vi "filter-scan-data-by-idx.vi"(9 "scan-idx-as-double":dbl=-1.0 format="%#_13g", 10 "meta-column-idx":i32=4, 11 "data-in":dbl[][](array[numeric])=[[1.0, 0.0, 0.0, 0.0, 1.0], [2.0, 0.0, 0.0, 0.0, 1.0], [3.0, 0.0, 0.0, 0.0, -1.0], [4.0, 0.0, 0.0, 0.0, -1.0], [5.0, 0.0, 0.0, 0.0, -1.0], [6.0, 0.0, 0.0, 0.0, -1.0], [7.0, 0.0, 0.0, 0.0, -1.0], [8.0, 0.0, 0.0, 0.0, -1.0], [9.0, 0.0, 0.0, 0.0, -1.0], [10.0, 0.0, 0.0, 0.0, 1.0], [11.0, 0.0, 0.0, 0.0, 4.0], [12.0, 0.0, 0.0, 0.0, 2.0], [13.0, 0.0, 0.0, 0.0, 1.0], [14.0, 10.0, 11.0, 12.0, -1.0]]) -> (3 "filtered-data":dbl[][](array[numeric]))   [LabVIEW 2017]
uses:
  <userlib>/_OpenG.lib/array/array.llb/Search 1D Array (DBL)__ogtk.vi
  <userlib>/_OpenG.lib/array/array.llb/Index 1D Array Elements (DBL)__ogtk.vi
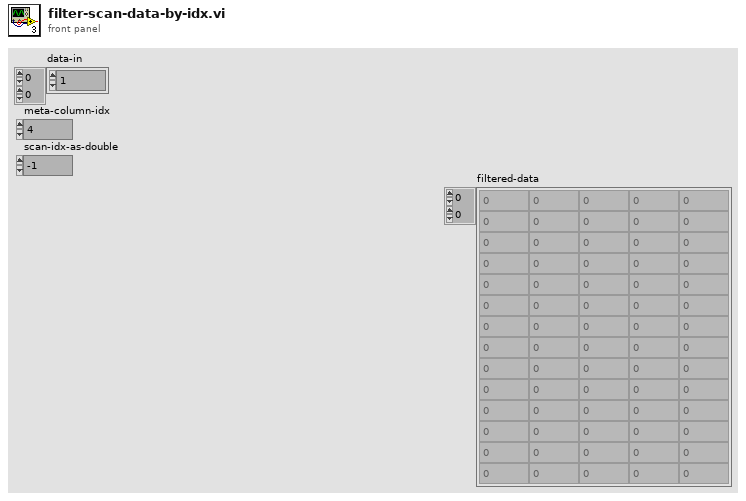
[diagram p1: front panel]
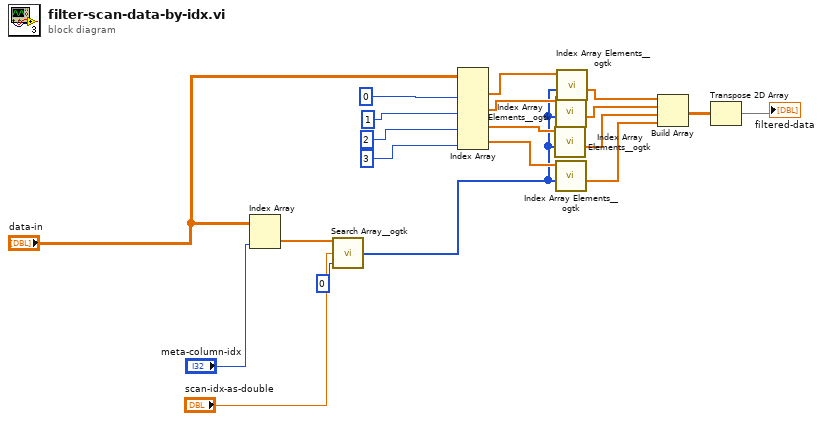
[diagram p0: block diagram]
diagram:
  n1 = Index Array(array="data-in", index (col)="meta-column-idx") -> (element=w19:dbl[])  [unwired: 1 in]
  n2 = call-poly <userlib>:"Search Array__ogtk.vi"("Array"=w19, "Element Data"="scan-idx-as-double", "Start Index (0)"=0) -> ("Indices of Elements"=w7:i32[])  [unwired: 6 in]
  n3 = Index Array(array="data-in", index (col) #1=0 ("disabled index (col)"), index (col) #2=1 ("disabled index (col)"), index (col) #3=2 ("disabled index (col)"), index (col) #4=3 ("disabled index (col)")) -> (element #1=w11:dbl[], element #2=w10:dbl[], element #3=w9:dbl[], element #4=w8:dbl[])  [unwired: 4 in]
  n4 = call-poly <userlib>:"Index Array Elements__ogtk.vi"("indices"=w7, "array"=w9) -> ("elements"=w4:dbl[])  [unwired: 9 in]
  n5 = call-poly <userlib>:"Index Array Elements__ogtk.vi"("indices"=w7, "array"=w10) -> ("elements"=w5:dbl[])  [unwired: 9 in]
  n6 = call-poly <userlib>:"Index Array Elements__ogtk.vi"("indices"=w7, "array"=w8) -> ("elements"=w3:dbl[])  [unwired: 9 in]
  n7 = call-poly <userlib>:"Index Array Elements__ogtk.vi"("indices"=w7, "array"=w11) -> ("elements"=w6:dbl[])  [unwired: 9 in]
  n8 = Build Array(w6, w5, w4, w3) -> (w2:dbl[][])
  n9 = Transpose 2D Array(2D array=w2) -> (transposed array=→"filtered-data":dbl[][])
